vi "FoCA.vi"() -> ()   [LabVIEW 2015]
panel:
  out "All files":path[](array[path])
  in  "current_curve":path
  out "active file name":string
  in  "data folder":path
  in  "data_type":enum16{"Nanopuller", "Agilent", "Bioscope"}(ring)
  in  "stop":bool
  in  "next":bool
  in  "prev":bool
  out "XY Graph":cluster{"X":dbl, "Y":dbl}[](graph)
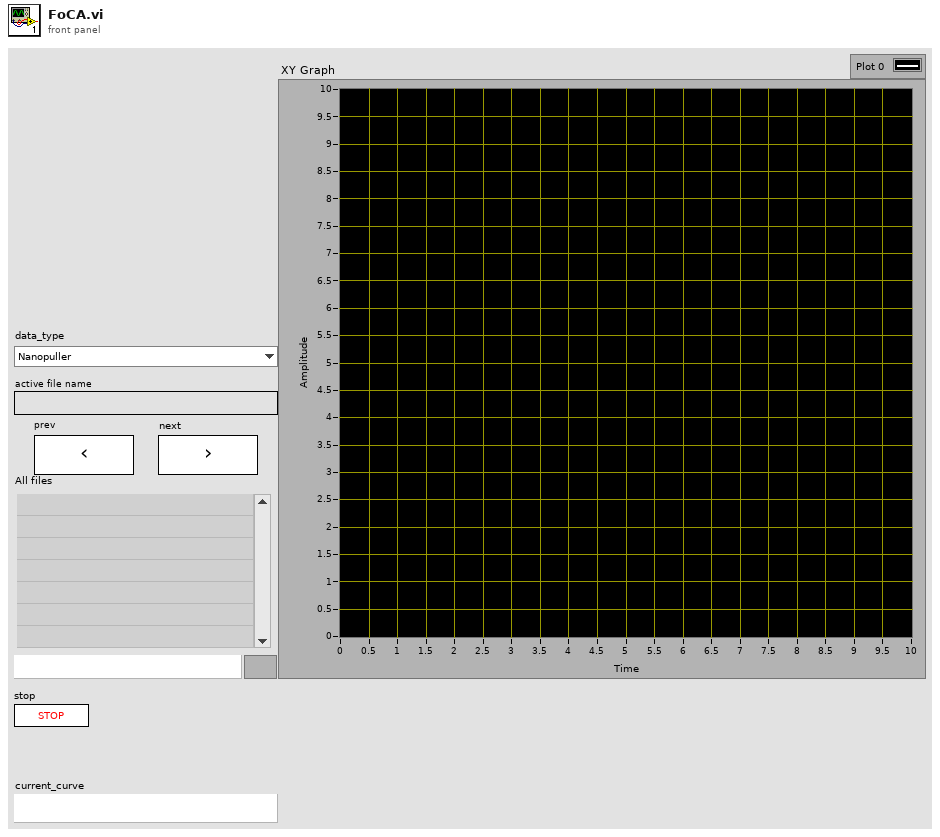
[diagram p1: front panel]
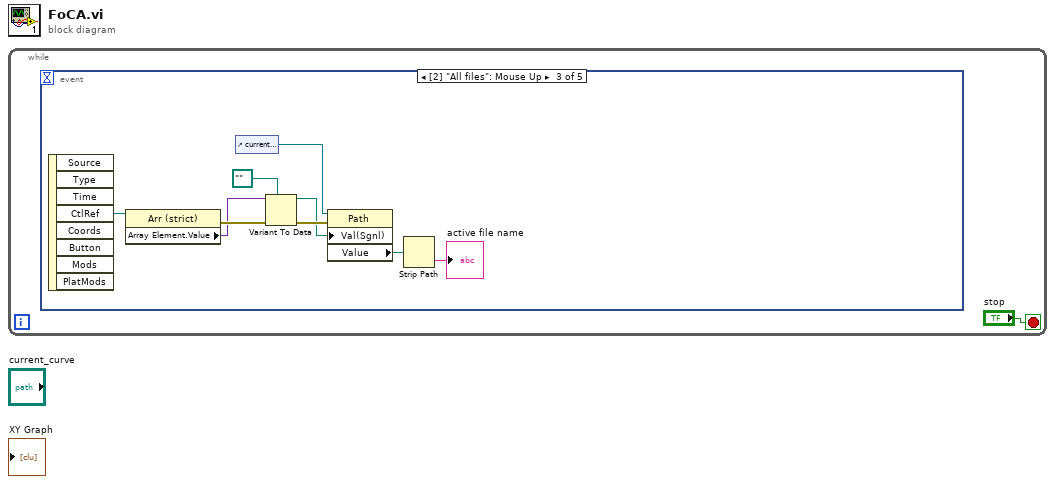
[diagram p0: block diagram]
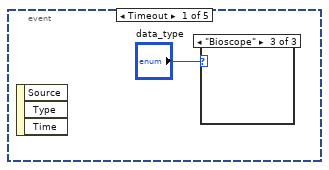
[diagram p2: hidden frame]
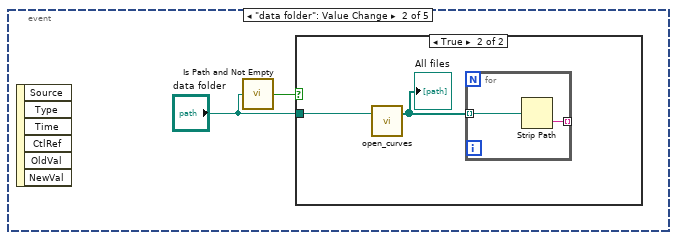
[diagram p5: hidden frame]
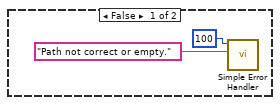
[diagram p6: hidden frame]
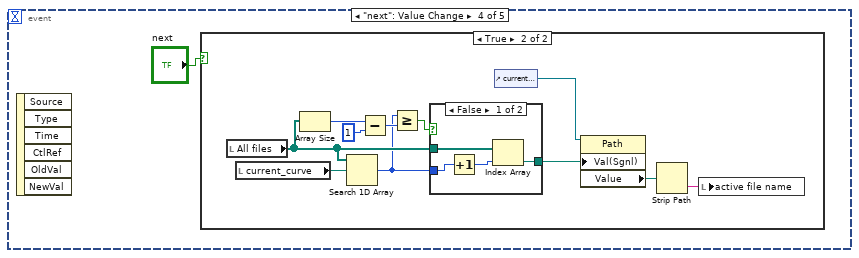
[diagram p7: hidden frame]
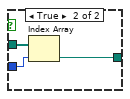
[diagram p9: hidden frame]
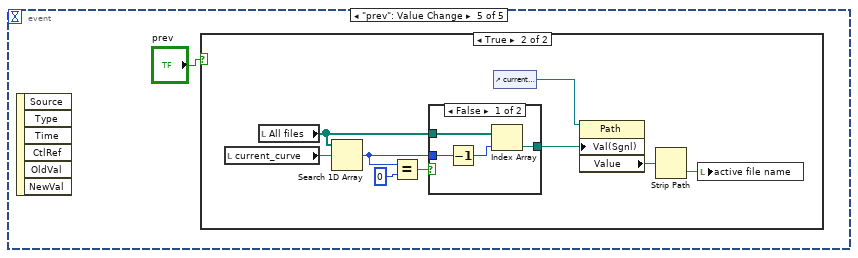
[diagram p10: hidden frame]
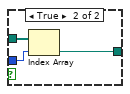
[diagram p12: hidden frame]
diagram:
  n1 = while {
    stop <- "stop" stop-if-true
    n2 = event shown="[2] \"All files\": Mouse Up" {
      selector: _ -> [_ _ _ _ _]
      dyn-events: _ -> [_ _ _ _ _]
      timeout: _ -> [_ _ _ _ _]
      event Timeout {
        n3 = event-data() -> ()  [unwired: 1 in, 3 out]
        n4 = case shown="\"Bioscope\"" "data_type" {
          frame "Nanopuller", Default {
          }
          frame "Agilent" {
          }
          frame "Bioscope" {
          }
        }
      }
      event "data folder": Value Change {
        n5 = event-data() -> ()  [unwired: 1 in, 6 out]
        n6 = call <vilib>:"Is Path and Not Empty.vi"("path"="data folder") -> ("Is Path and Not Empty?"=w4:bool)  [unwired: 4 in]
        n7 = case shown="True" w4 {
          tunnel: "data folder" -> [_ w8]
          frame False {
            n8 = call <vilib>:"Simple Error Handler.vi"("error code (no error:0)"=100, "error source (\" \")"="Path not correct or empty." ("error source (\" \")")) -> ()  [unwired: 3 in, 5 out]
          }
          frame True {
            n9 = call "open_curves.vi"("Path"=w8) -> ("All TXT files"=w7:path[])  [unwired: 1 in, 1 out]
            "All files" <- w7
            n10 = for {
              tunnel: w7 -> [w10] mode=indexing
              tunnel: [w9] -> _ mode=indexing
              n11 = Strip Path(path=w10) -> (name=w9:string)  [unwired: 1 out]
            }
          }
        }
      }
      event "All files": Mouse Up {
        n12 = event-data() -> ("CtlRef"=w11:refnum<vi>)  [unwired: 1 in, 7 out]
        n13 = property class="Arr (strict)"(reference=w11) -> (error out=w18:errorcluster, "Array Element.Value"=w15:variant)  [unwired: 1 in, 1 out]
        n14 = control-ref of="current_curve"() -> (w16:refnum<vi>)
        n15 = Variant To Data(error in=w18, type=path "", Variant=w15) -> (data=w17:path, error out=w19:errorcluster)
        n16 = property class="Path"(reference=w16, error in=w19, "Val(Sgnl)"=w17) -> ("Value"=w13:path)  [unwired: 2 out]
        n17 = Strip Path(path=w13) -> (name=→"active file name":string)  [unwired: 1 out]
      }
      event "next": Value Change {
        n18 = event-data() -> ()  [unwired: 1 in, 6 out]
        n19 = case shown="True" "next" {
          frame False {
          }
          frame True {
            n20 = local read "All files"() -> (w27:path[])
            n21 = local read "current_curve"() -> (w24:path)
            n22 = Array Size(array=w27) -> (size(s)=w29:i32)
            n23 = Search 1D Array(1D array=w27, element=w24) -> (index of element=w25:i32)  [unwired: 1 in]
            n24 = Subtract(x=w29, y=1) -> (x-y=w31:i32)
            n25 = Greater Or Equal?(x=w25, y=w31) -> (x >= y?=w28:bool)
            n26 = case shown="False" w28 {
              tunnel: w25 -> [w34 w38]
              tunnel: w27 -> [w33 w37]
              tunnel: [w32 w36] -> w26
              frame False {
                n27 = Increment(x=w34) -> (x+1=w35:i32)
                n28 = Index Array(array=w33, index=w35) -> (element=w32:path)
              }
              frame True {
                n29 = Index Array(array=w37, index=w38) -> (element=w36:path)
              }
            }
            n30 = control-ref of="current_curve"() -> (w23:refnum<vi>)
            n31 = property class="Path"(reference=w23, "Val(Sgnl)"=w26) -> ("Value"=w21:path)  [unwired: 1 in, 2 out]
            n32 = Strip Path(path=w21) -> (name=w22:string)  [unwired: 1 out]
            n33 = local write "active file name"(w22) -> ()
          }
        }
      }
      event "prev": Value Change {
        n34 = event-data() -> ()  [unwired: 1 in, 6 out]
        n35 = case shown="True" "prev" {
          frame False {
          }
          frame True {
            n36 = local read "current_curve"() -> (w48:path)
            n37 = local read "All files"() -> (w45:path[])
            n38 = Search 1D Array(1D array=w45, element=w48) -> (index of element=w47:i32)  [unwired: 1 in]
            n39 = Equal?(x=w47, y=0) -> (x = y?=w44:bool)
            n40 = case shown="False" w44 {
              tunnel: w47 -> [w51 w55]
              tunnel: w45 -> [w50 w54]
              tunnel: [w49 w53] -> w46
              frame False {
                n41 = Decrement(x=w51) -> (x-1=w52:i32)
                n42 = Index Array(array=w50, index=w52) -> (element=w49:path)
              }
              frame True {
                n43 = Index Array(array=w54, index=w55) -> (element=w53:path)
              }
            }
            n44 = control-ref of="current_curve"() -> (w42:refnum<vi>)
            n45 = property class="Path"(reference=w42, "Val(Sgnl)"=w46) -> ("Value"=w40:path)  [unwired: 1 in, 2 out]
            n46 = Strip Path(path=w40) -> (name=w41:string)  [unwired: 1 out]
            n47 = local write "active file name"(w41) -> ()
          }
        }
      }
    }
  }
